vi "PXI MAC Address.vi"() -> (1 "Current PXI Chassis":string=" unknown")   [LabVIEW 2015]
doc: "revised 2010Feb8 fsc [no longer calls .dll ]\n\n\nThis VI calls MACaddress.dll to get the first MAC address of the current computer, and compare it with the MAC addresses of the chambers set by the user.\nTo get MAC address in Windows:\nGo to Start->run, type in \"cmd\", a console window will pop up. Then type \"ipconfig/all\", the information after \"Physical Address\" is the MAC address . Copy that number and please remember to REMOVE THE DASHES.\n-- 12/2004 Haobing Wang"
panel:
  in  "PXI MAC Address Array":cluster{string, string}[](array[cluster])=[{"Ch4b pxi dual", "00-80-2F-10-BE-2F"}, {"Ch4A pxi quad", "00-80-2F-11-E3-F4"}, {"Ch411 pxi dual", "00-80-2F-A-9F-DE"}, {" ABI pxi dual", "00-80-2F-10-BB-AC"}, {"Ch2 pxi quad", "00-80-2F-11-E4-1"}, {"Ch2 pxi quad", "00-80-2F-0A-A2-33"}, {" Ch2 pxi dual", "00-80-2F-A-9F-EC"}, {" engr-pxi-quad", "00-80-2F-11-E4-3"}, {" engr-pxi-quad", "00-80-2F-0A-A2-28"}, {" Shera pxi quad", "00-80-2F-11-E3-F5"}, {" Ch3a pxi Dual", "00-80-2F-11-E4-9"}, {" Ch3a pxi Quad", "00-80-2F-10-A9-3C"}, {" Ch3a pxi Quad", "00-80-2F-0A-5E-35"}, {"Ch3b pxi Dual", "00-80-2F-11-E3-F8"}, {"Ch3b pxi Quad", "00-80-2F-10-85-73"}, {"Ch3b pxi Quad", "00-80-2F-0A-96-14"}, {"Ch3a Vital Signs pxi", "00-80-2F-0A-96-EC"}, {" Sewell pxi Dual", "00-80-2F-10-BE-E3"}, {" Polley pxi Quad", "00-80-2F-11-E4-2"}, {" Shera pxi dual", "00-80-2F-10-EB-60"}, {"", ""}]
  out "MAC Address of currentPXI Chassis":string="00-80-2F-0A-A2-28"
  # "modified 2010 FEB 08 fsc to use a system cmd instead of .dll. \n\nTo get MAC address in Windows:\nGo to Start->run, type in \"cmd\", a console window will pop up. Then type \"ipconfig/all\", the information after \"Physical Address\" is the MAC address . \n-- 12/2004 Haobing Wang"
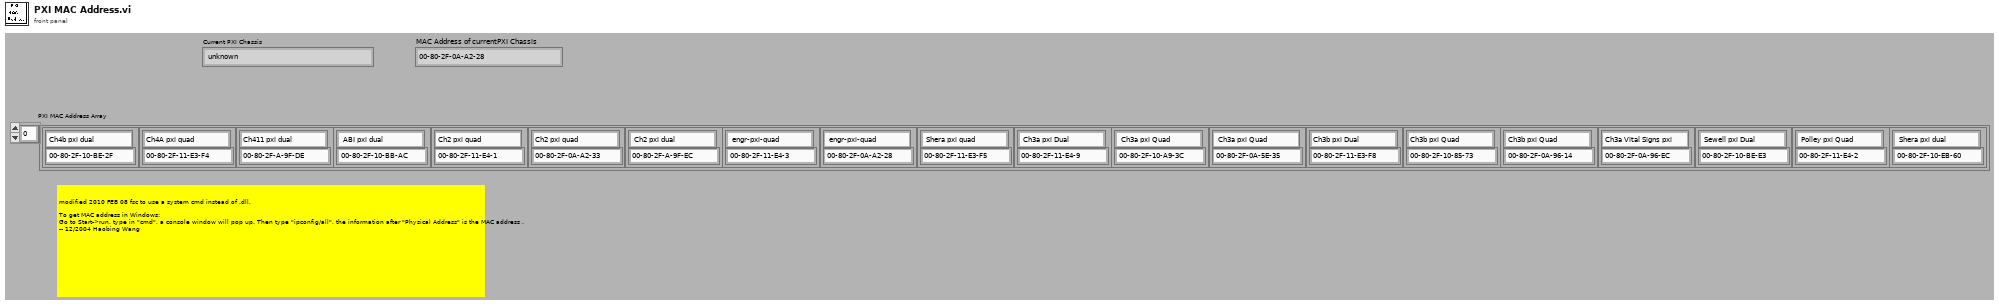
[diagram p1: front panel]
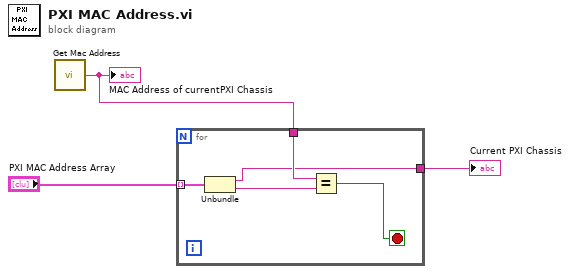
[diagram p0: block diagram]
diagram:
  n1 = call "Get Mac Address.vi"() -> ("MAC Address"=w2:string)  [unwired: 5 in]
  "MAC Address of currentPXI Chassis" <- w2
  n2 = for {
    tunnel: "PXI MAC Address Array" -> [w8] mode=indexing
    tunnel: w2 -> [w6]
    tunnel: [w4] -> w1
    stop <- w5 stop-if-true
    n3 = Unbundle(w8) -> (w4:string, w7:string)
    n4 = Equal?(x=w6, y=w7) -> (x = y?=w5:bool)
  }
  "Current PXI Chassis" <- w1
